vi "Motion Plot sub_VI.vi"(8 "Motion Parameters":T2={"Decel Time (s)"=0.0, "Accel Time (s)"=0.0, "Total Time (s)"=0.0, "Accel (mm/s^2)"=0.0, "Decel (mm/s^2)"=0.0, "Time step (s)"=0.01} {"Time step (s)" min=0.001}) -> (0 "Motion Points":T1, 1 "Accel Array 2":dbl[](graph), 2 "Velocity Array 2":dbl[](graph), 3 "Displacement Array 2":dbl[](graph), 4 "V max (mm/s)":dbl, 5 "Dist max (mm)":dbl)   [LabVIEW 2017]
uses:
  <vilib>/imath/engines/lvmath2/RunTimeEngine/BuiltInFunctions/round/NIMS_round(DBL-S).vi
  <vilib>/imath/engines/lvmath2/RunTimeEngine/BuiltInFunctions/zeros/NIMS_V=zeros(I32,I32).vi
  <vilib>/imathl/engines/lvmath/Functions/Error Handling/Create Error.vi
  <vilib>/imath/engines/lvmath2/RunTimeEngine/IndexReplace/NIMS V(S)=S.vi
  <instcachedir>/0/NIMS V(S)=S_3F4D177D41884A9C969E5FA0B22E4B28.lvgen/NIMS V(S)=S_3F4D177D41884A9C969E5FA0B22E4B28_003.vi
  <instcachedir>/0/NIMS V(S)=S_3F4D177D41884A9C969E5FA0B22E4B28.lvgen/NIMS V(S)=S_3F4D177D41884A9C969E5FA0B22E4B28_000.vi
  <vilib>/imath/engines/lvmath2/RunTimeEngine/RangeToken/NIMS_Range_R2 - Float.vi
  <instcachedir>/0/NIMS_Range_R2 - Float_6729C30523D247ACAEE4609355DED762.lvgen/NIMS_Range_R2 - Float_6729C30523D247ACAEE4609355DED762_000.vi
  <vilib>/imath/engines/lvmath2/RunTimeEngine/CommandStatement/MC_CommandStatement_break.vi
  <vilib>/imath/engines/lvmath2/RunTimeSupport/NIMS_Error if Not Equal.vi
  <instcachedir>/0/NIMS_Error if Not Equal_6374CBDCC5AA461FB337545605D07630.lvgen/NIMS_Error if Not Equal_6374CBDCC5AA461FB337545605D07630_000.vi
  <vilib>/imath/engines/lvmath2/RunTimeEngine/ErrorHandling/NIMS_Create Error From Enums.vi
  <vilib>/imath/engines/lvmath2/RunTimeEngine/IndexRead/NIMS V(S).vi
  <instcachedir>/0/NIMS V(S)_0488751826AF41519A22953C041130DC.lvgen/NIMS V(S)_0488751826AF41519A22953C041130DC_000.vi
  <vilib>/imath/engines/lvmath2/RunTimeEngine/NodeEndStatement/NIMS_NodeEndStatement_Output.vi
  <instcachedir>/0/NIMS_NodeEndStatement_Output_53EC0D466D134D7ABD903AC30B43404B.lvgen/NIMS_NodeEndStatement_Output_53EC0D466D134D7ABD903AC30B43404B_005.vi
  <vilib>/imath/engines/lvmath2/RunTimeEngine/ErrorHandling/NIMS_Finalize Error.vi
panel:
  # "Use 0.01s"
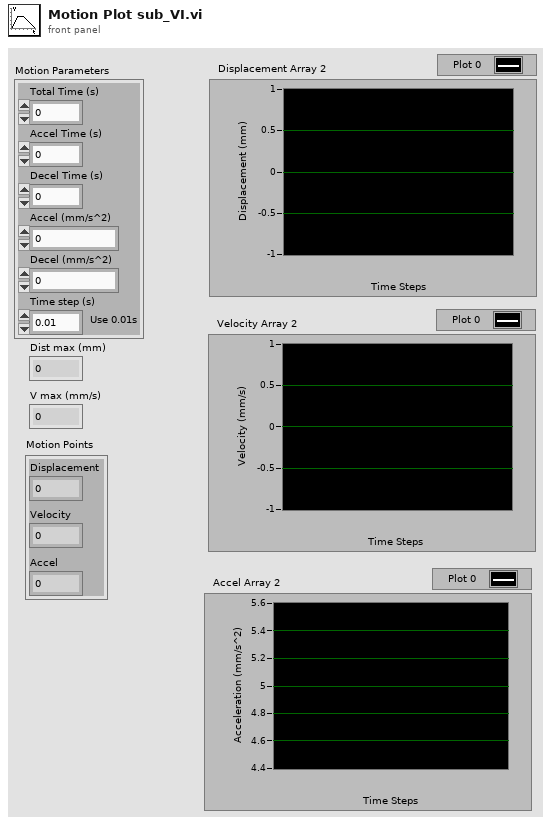
[diagram p1: front panel]
types:
  T1 = cluster{"Accel":dbl, "Velocity":dbl, "Displacement":dbl}
  T2 = cluster{"Decel Time (s)":dbl, "Accel Time (s)":dbl, "Total Time (s)":dbl, "Accel (mm/s^2)":dbl, "Decel (mm/s^2)":dbl, "Time step (s)":dbl}
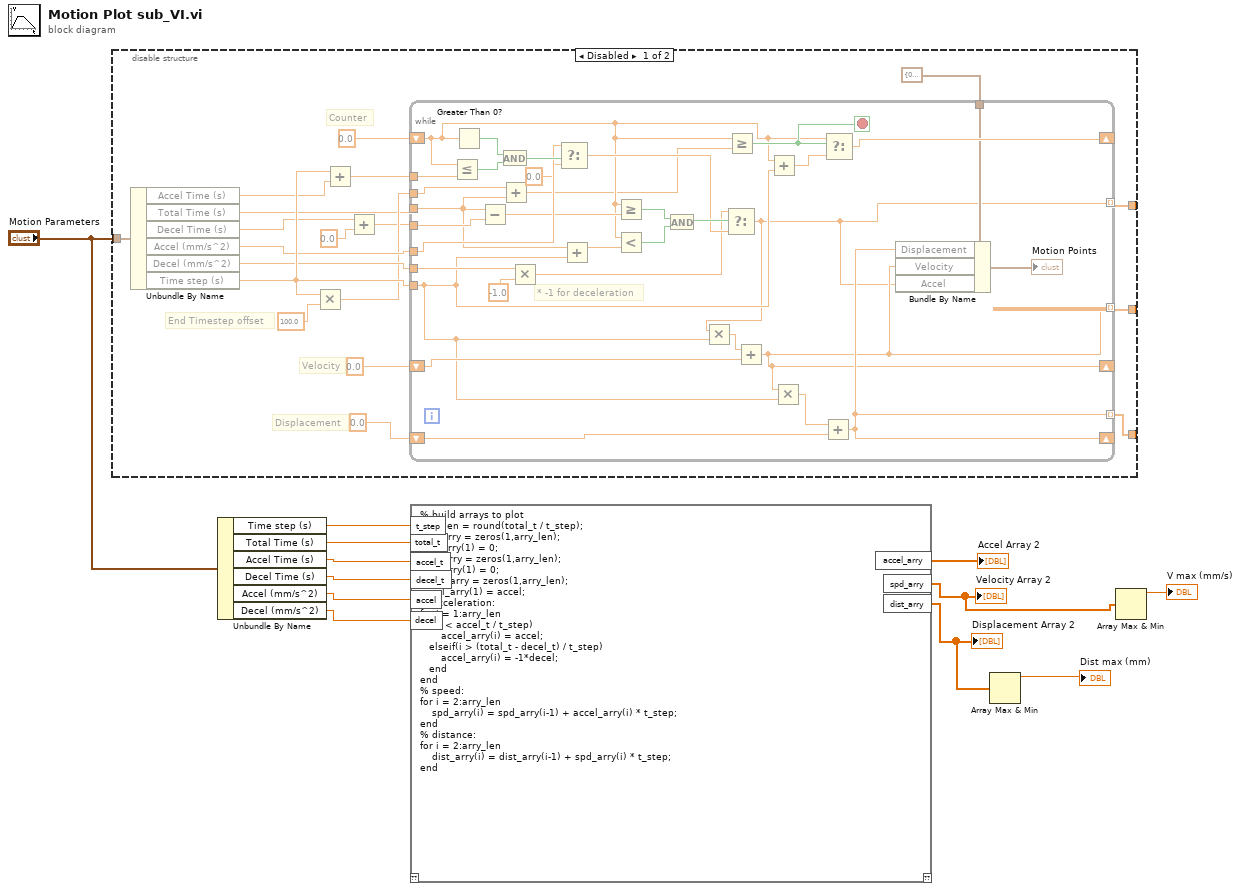
[diagram p0: block diagram]
diagram:
  n1 = disable-structure shown="Disabled" {
    disable-tunnel: "Motion Parameters" -> [w31 _]
    disable-tunnel: [w30 _] -> _
    disable-tunnel: [w17 _] -> _
    disable-tunnel: [w14 _] -> _
    frame Disabled {
      # "End Timestep offset"
      # "Displacement"
      # "Velocity"
      # "Counter"
      n2 = Unbundle By Name(w31) -> ("Accel Time (s)"=w15:dbl, "Total Time (s)"=w16:dbl, "Decel Time (s)"=w18:dbl, "Accel (mm/s^2)"=w27:dbl, "Decel (mm/s^2)"=w28:dbl, "Time step (s)"=w29:dbl)
      n3 = Multiply(x=w29, y=100.0) -> (x*y=w26:dbl)
      n4 = Add(x=w29, y=w15) -> (x+y=w22:dbl)
      n5 = Add(x=w18, y=0.0) -> (x+y=w23:dbl)
      n6 = while {
        shift-right: [w42] -> _
        shift-left: 0.0 -> [w41]
        tunnel: w22 -> [w64]
        tunnel: w27 -> [w60]
        tunnel: w16 -> [w52]
        tunnel: w23 -> [w57]
        tunnel: [w32] -> w17 mode=indexing
        tunnel: w28 -> [w44]
        shift-right: [w33] -> _
        shift-left: 0.0 -> [w49]
        shift-right: [w36] -> _
        shift-left: 0.0 -> [w47]
        tunnel: [w33] -> w30 mode=indexing
        tunnel: [w36] -> w14 mode=indexing
        tunnel: w29 -> [w39]
        tunnel: w26 -> [w37]
        tunnel: T1 {"Accel"=0.0, "Velocity"=0.0, "Displacement"=0.0} ("Motion Points 2") -> [w34]
        stop <- w50 stop-if-true
        # "* -1 for deceleration"
        n7 = Less Or Equal?(x=w41, y=w64) -> (x <= y?=w62:bool)
        n8 = Greater Than 0?(x=w41) -> (x > 0?=w63:bool)
        n9 = Subtract(x=w52, y=w57) -> (x-y=w58:dbl)
        n10 = And(x=w63, y=w62) -> (x .and. y?=w61:bool)
        n11 = Add(x=w37, y=w52) -> (x+y=w38:dbl)
        n12 = Multiply(x=w44, y=-1.0 ("x")) -> (x*y=w45:dbl)
        n13 = Select(t=w60, s=w61, f=0.0) -> (s? t:f=w53:dbl)
        n14 = Add(x=w52, y=w39) -> (x+y=w40:dbl)
        n15 = Greater Or Equal?(x=w41, y=w58) -> (x >= y?=w56:bool)
        n16 = Less?(x=w41, y=w40) -> (x < y?=w55:bool)
        n17 = And(x=w56, y=w55) -> (x .and. y?=w54:bool)
        n18 = Select(t=w45, s=w54, f=w53) -> (s? t:f=w32:dbl)
        n19 = Multiply(x=w32, y=w39) -> (x*y=w48:dbl)
        n20 = Greater Or Equal?(x=w41, y=w38) -> (x >= y?=w50:bool)
        n21 = Add(x=w48, y=w49) -> (x+y=w33:dbl)
        n22 = Add(x=w41, y=w39) -> (x+y=w51:dbl)
        n23 = Multiply(x=w33, y=w39) -> (x*y=w46:dbl)
        n24 = Add(x=w46, y=w47) -> (x+y=w36:dbl)
        n25 = Select(t=w41, s=w50, f=w51) -> (s? t:f=w42:dbl)
        n26 = Bundle By Name(cluster=w34, "Displacement"=w36, "Velocity"=w33, "Accel"=w32) -> (→"Motion Points":T1)
      }
    }
    frame Enabled {
    }
  }
  n27 = Unbundle By Name("Motion Parameters") -> ("Time step (s)"=w11:dbl, "Total Time (s)"=w10:dbl, "Accel Time (s)"=w9:dbl, "Decel Time (s)"=w8:dbl, "Accel (mm/s^2)"=w7:dbl, "Decel (mm/s^2)"=w6:dbl)
  n28 = mathscript code="% build arrays to plot\narry_len = round(total_t / t_step);\nspd_arry = zeros(1,arry_len);\nspd_arry(1) = 0;\ndist_arry = zeros(1,arry_len);\ndist_arry(1) = 0;\naccel_arry = zeros(1,arry_len);\naccel_arry(1) = accel;\n% acceleration:\nfor i = 1:arry_len\n   if(i < accel_t / t_step)\n       accel_arry(i) = accel;\n   elseif(i > (total_t - decel_t) / t_step)\n       accel_arry(i) = -1*decel;\n   end\nend\n% speed:\nfor i = 2:arry_len\n    spd_arry(i) = spd_arry(i-1) + accel_arry(i) * t_step;\nend\n% distance:\nfor i = 2:arry_len\n    dist_arry(i) = dist_arry(i-1) + spd_arry(i) * t_step;\nend"("total_t"=w10, "t_step"=w11, "accel_t"=w9, "decel_t"=w8, "accel"=w7, "decel"=w6) -> ("accel_arry"=→"Accel Array 2":dbl[], "spd_arry"=w1:dbl[], "dist_arry"=w4:dbl[])  [unwired: 1 in, 1 out]
  "Velocity Array 2" <- w1
  "Displacement Array 2" <- w4
  n29 = Array Max & Min(array=w4) -> (max value=→"Dist max (mm)":dbl)  [unwired: 3 out]
  n30 = Array Max & Min(array=w1) -> (max value=→"V max (mm/s)":dbl)  [unwired: 3 out]
